vi "Write Topic Filter.vi"(10 "Topic Filter":string, 11 "TopicFilter in":refnum<class "TopicFilter.lvclass">) -> (3 "TopicFilter out":refnum<class "TopicFilter.lvclass">)   [LabVIEW 2013, in "MQTT Server.lvlib" / "TopicFilter.lvclass"]
uses:
  TopicFilter.lvclass
  TopicFilter.lvclass/TopicFilter.ctl
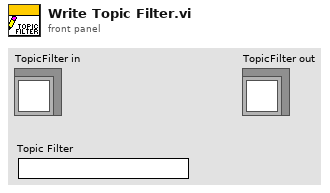
[diagram p1: front panel]
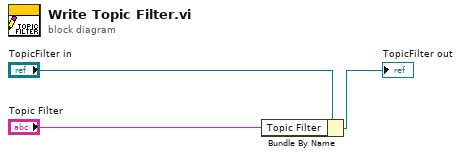
[diagram p0: block diagram]
diagram:
  n1 = Bundle By Name(cluster="TopicFilter in", "Topic Filter"="Topic Filter") -> (→"TopicFilter out":refnum<class "TopicFilter.lvclass">)
